vi "Update Status List.vi"(8 "error in (no error)":errorcluster, 10 "Status List":string[](array[string]), 11 "Chat Window Interface in":refnum<class "Chat Window Interface.lvclass">) -> (0 "error out":errorcluster, 3 "Chat Window Interface out":refnum<class "Chat Window Interface.lvclass">)   [LabVIEW 2015, in "Chat Window Interface.lvlib" / "Chat Window Interface.lvclass"]
uses:
  Chat Window Interface.lvclass
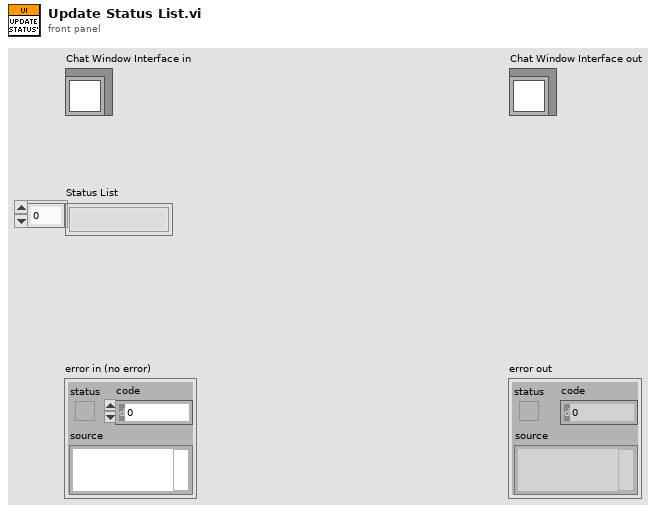
[diagram p1: front panel]
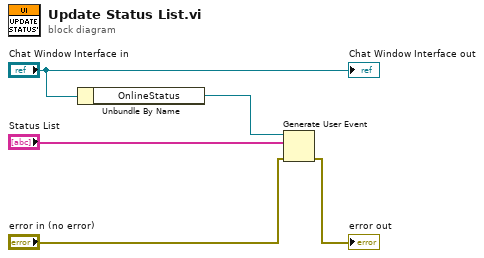
[diagram p0: block diagram]
diagram:
  n1 = Unbundle By Name("Chat Window Interface in") -> ("OnlineStatus"=w4:refnum<user-event>)
  n2 = Generate User Event(user event=w4, event data cluster="Status List", error in="error in (no error)") -> (error out=→"error out":errorcluster)  [unwired: 1 in, 1 out]
  "Chat Window Interface out" <- "Chat Window Interface in"
